vi "VWflipper.vi"(7 "Theta Degree":dbl, 8 "Probe w m/s":dbl, 9 "Probe v m/s":dbl, 10 "Probe u  m/s":dbl, 11 "VMagn m/s":dbl) -> (3 "VmagUVWCone":dbl[](array[numeric]))   [LabVIEW 2013]
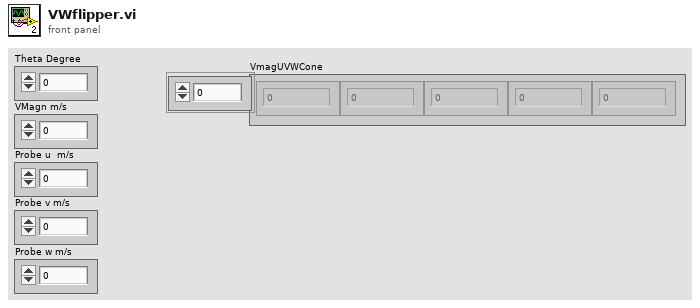
[diagram p1: front panel]
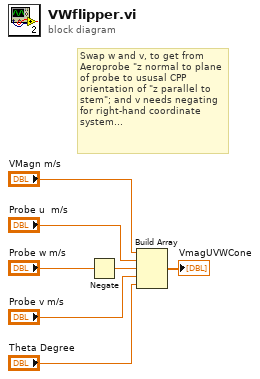
[diagram p0: block diagram]
diagram:
  # "Swap w and v, to get from Aeroprobe \"z normal to plane of probe to ususal CPP orientation of \"z parallel to stem\"; and v needs negating for right-hand coordinate system..."
  n1 = Negate(x="Probe w m/s") -> (-x=w3:dbl)
  n2 = Build Array("VMagn m/s", "Probe u  m/s", w3, "Probe v m/s", "Theta Degree") -> (→"VmagUVWCone":dbl[])
